vi "Load All Categories.vi"(8 "error in (no error)":errorcluster, 11 "Budgetizer in":refnum<class "Budgetizer.lvclass">) -> (0 "error out":errorcluster, 2 "Categories":refnum<class "Category.lvclass">[](array[class]), 3 "Budgetizer out":refnum<class "Budgetizer.lvclass">)   [LabVIEW 2018, in "Budgetizer.lvclass"]
uses:
  Budgetizer.lvclass
  Category/Category.lvclass
  Budgetizer.lvclass/Budgetizer.ctl
  database/Database.lvclass
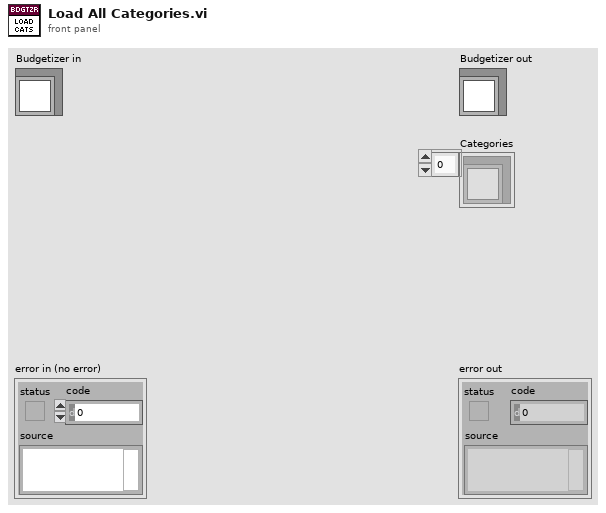
[diagram p1: front panel]
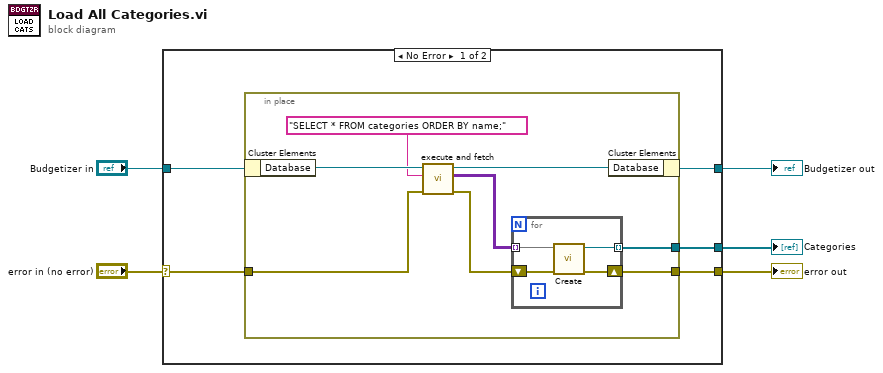
[diagram p0: block diagram]
diagram:
  n1 = case shown="No Error" "error in (no error)" {
    selector: "error in (no error)" -> [w7 w24]
    tunnel: [w8 w24] -> w4
    tunnel: [w9 w23] -> w2
    tunnel: "Budgetizer in" -> [w10 w23]
    tunnel: [w6 _] -> w1
    frame No Error {
      n2 = in-place {
        in-place-border: w7 -> [w16]
        in-place-border: [w12] -> w8
        in-place-border: [w11] -> w6
        n3 = in-place-cluster #1(w10) -> ("Database"=w18:refnum<class "Database.lvclass">)
        n4 = call "execute and fetch.vi"("error in (no error)"=w16, "SQL query"="SELECT * FROM categories ORDER BY name;", "Database in"=w18) -> ("error out"=w13:errorcluster, "recordset data"=w14:variant[][], "Database out"=w17:refnum<class "Database.lvclass">)  [unwired: 5 in, 1 out]
        n5 = for {
          tunnel: w14 -> [w22] mode=indexing
          shift-right: [w19] -> w12
          shift-left: w13 -> [w21]
          tunnel: [w20] -> w11 mode=indexing
          n6 = call "Create.vi"("error in (no error)"=w21, "Record"=w22) -> ("error out"=w19:errorcluster, "Category out"=w20:refnum<class "Category.lvclass">)  [unwired: 8 in]
        }
        n7 = in-place-cluster #1("Database"=w17) -> (w9:refnum<class "Budgetizer.lvclass">)
      }
    }
    frame Error {
    }
  }
  "error out" <- w4
  "Budgetizer out" <- w2
  "Categories" <- w1
